vi "Version.vi"(8 "error in (no error)":errorcluster) -> (0 "error out":errorcluster, 1 "Minor":i32, 2 "Major":i32, 3 "Version String":string, 4 "Fix":i32)   [LabVIEW 2015]
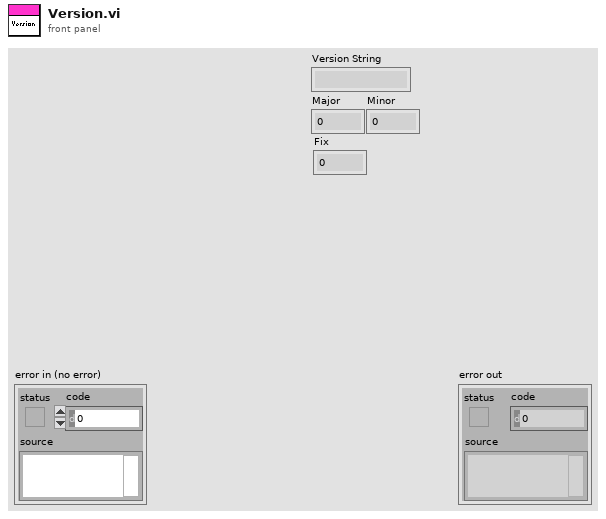
[diagram p1: front panel]
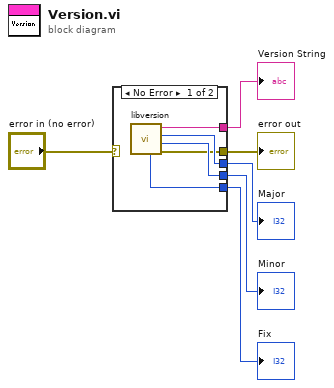
[diagram p0: block diagram]
diagram:
  n1 = case shown="No Error" "error in (no error)" {
    selector: "error in (no error)" -> [_ w12]
    tunnel: [w8 w12] -> w5
    tunnel: [w11 _] -> w4
    tunnel: [w10 _] -> w3
    tunnel: [w9 _] -> w2
    tunnel: [w7 _] -> w1
    frame No Error {
      n2 = call "libversion.vi"() -> ("error out"=w8:errorcluster, "Minor"=w9:i32, "Major"=w10:i32, "Version String"=w11:string, "Fix"=w7:i32)  [unwired: 7 in]
    }
    frame Error {
    }
  }
  "error out" <- w5
  "Version String" <- w4
  "Minor" <- w2
  "Fix" <- w1
  "Major" <- w3
